vi "dfd_Get Folder Name.vi"(10 "filter name":string) -> (1 "folder name":string, 2 "dup filter name":string)   [LabVIEW 2017, in "NI_DigFilterLicensed.lvlib"]
uses:
  <vilib>/addons/Digital Filter Design/NI_DigFilterLicensed.lvlib
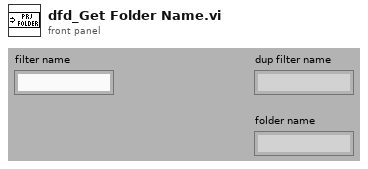
[diagram p1: front panel]
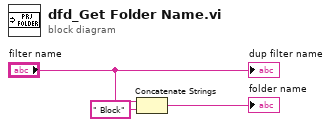
[diagram p0: block diagram]
diagram:
  n1 = Concatenate Strings("filter name", " Block" ("string")) -> (→"folder name":string)
  "dup filter name" <- "filter name"
